vi "CL3IF_ResetGroup.vi"(7 "group":T1 items=["GROUP1"=1, "GROUP2"=2], 8 "error in":errorcluster {"code" format="%x"}, 11 "deviceId":i32) -> (0 "error out":errorcluster {"code" format="%x"})   [LabVIEW 2020, in "Keyence CL-3000.lvlib"]
doc: "This function resets the OUT group set with terminal allocation."
uses:
  Keyence CL-3000.lvlib
  enums/CL3IF_RESET_GROUP.ctl
  Private/enums/Function Name.ctl
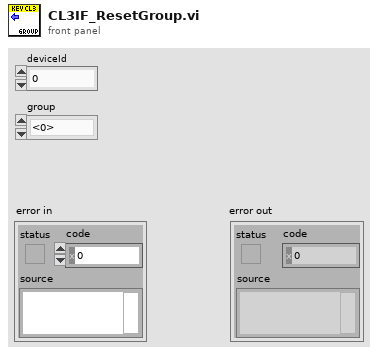
[diagram p1: front panel]
types:
  T1 = typedef "Keyence CL-3000.lvlib/CL3IF_RESET_GROUP.ctl" = u16
  T2 = typedef "Keyence CL-3000.lvlib/Function Name.ctl" = enum16{"Initialize", "Close", "CL3IF_GetMeasurementData", "CL3IF_GetTrendIndex", "CL3IF_GetTrendData", "CL3IF_GetStorageIndex", "CL3IF_GetStorageData", "CL3IF_AutoZeroMulti", "CL3IF_AutoZeroGroup", "CL3IF_TimingMulti", "CL3IF_TimingGroup", "CL3IF_ResetMulti", "CL3IF_ResetGroup", "CL3IF_LightControl", "CL3IF_MeasurementControl", "CL3IF_SwitchProgram", "CL3IF_GetProgramNo", "CL3IF_StartStorage", "CL3IF_StopStorage", "CL3IF_ClearStorageData", "CL3IF_GetPulseCount", "CL3IF_ResetPulseCount", "CL3IF_GetLightWaveform"}
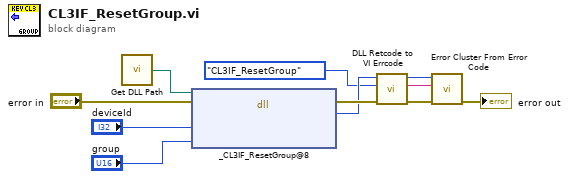
[diagram p0: block diagram]
diagram:
  n1 = call "Get DLL Path.vi"() -> ("DLL Path"=w8:path)  [unwired: 1 in]
  n2 = dll-call lib="C:/Program Files (x86)/National Instruments/LabVIEW 2018/instr.lib/Keyence CL-3000/CL3_IF.dll" fn="_CL3IF_ResetGroup@8"(path in=w8, error in="error in", "deviceId"="deviceId", "group"="group") -> (error out=w6:errorcluster, "RC"=w5:i32)  [unwired: 3 in, 1 out]
  n3 = call "DLL Retcode to VI Errcode.vi"("error in (no error)"=w6, "Function Name"=Function_Name."CL3IF_ResetGroup", "DLL Retcode"=w5) -> ("error out"=w11:errorcluster, "ErrorMessage"=w2:string, "VI Errcode"=w10:i32)  [unwired: 6 in]
  n4 = call <vilib>:"Error Cluster From Error Code.vi"("error in (no error)"=w11, "error message (\"\")"=w2, "error code (0)"=w10) -> ("error out"=→"error out":errorcluster)  [unwired: 6 in]
